vi "RestartIfDisconnected.vi"(8 "error in (no error)":errorcluster, 9 "connection timeout":i32=-1, 11 "NetworkStreamReader in":refnum<class "NetworkStreamReader.lvclass">) -> (0 "error out":errorcluster, 3 "NetworkStreamReader out":refnum<class "NetworkStreamReader.lvclass">)   [LabVIEW 2011, in "NetworkStreamReader.lvclass"]
uses:
  NetworkStreamReader.lvclass
  NetworkStreamReader.lvclass/NetworkStreamReader.ctl
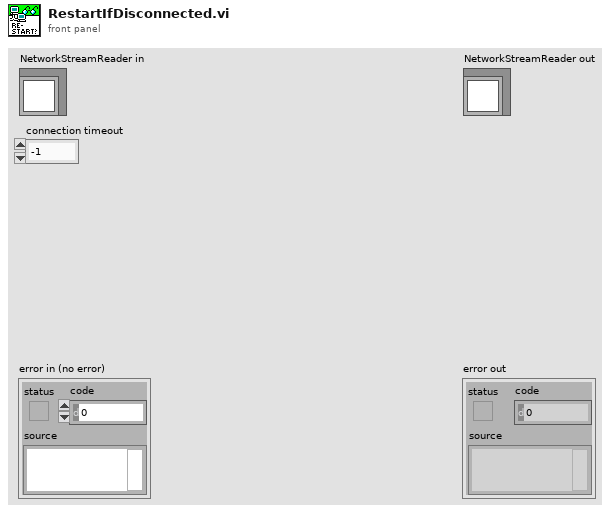
[diagram p1: front panel]
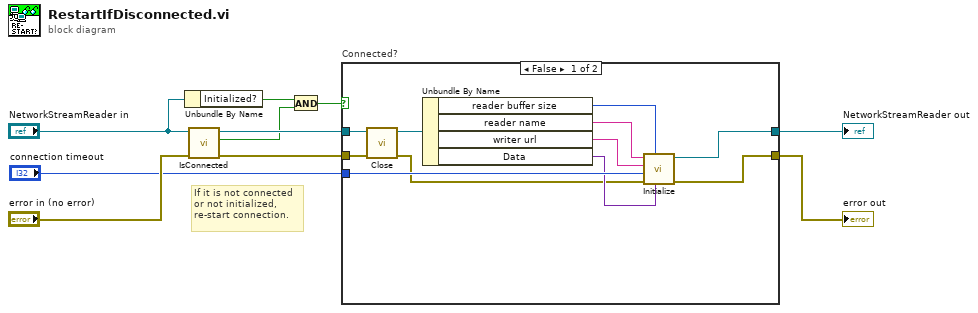
[diagram p0: block diagram]
diagram:
  # "If it is not connected\nor not initialized,\nre-start connection."
  n1 = Unbundle By Name("NetworkStreamReader in") -> ("Initialized?"=w2:bool)
  n2 = call "IsConnected.vi"("error in (no error)"="error in (no error)", "NetworkStreamReader in"="NetworkStreamReader in") -> ("error out"=w4:errorcluster, "Connected?"=w1:bool, "NetworkStreamReader out"=w5:refnum<class "NetworkStreamReader.lvclass">)  [unwired: 7 in]
  n3 = And(x=w2, y=w1) -> (x .and. y?=w3:bool)
  n4 = case "Connected?" shown="False" w3 {
    tunnel: w5 -> [w19 w23]
    tunnel: w4 -> [w18 w22]
    tunnel: [w12 w23] -> w7
    tunnel: [w11 w22] -> w9
    tunnel: "connection timeout" -> [w21 _]
    frame False {
      n5 = call "Close.vi"("error in (no error)"=w18, "NetworkStreamReader in"=w19) -> ("error out"=w13:errorcluster, "NetworkStreamReader out"=w17:refnum<class "NetworkStreamReader.lvclass">)  [unwired: 8 in]
      n6 = Unbundle By Name(w17) -> ("reader buffer size"=w20:i32, "reader name"=w16:string, "writer url"=w15:string, "Data"=w14:variant)
      n7 = call "Initialize.vi"("Default return"=w14, "reader buffer size"=w20, "error in (no error)"=w13, "connection timeout"=w21, "writer url"=w15, "reader name"=w16) -> ("error out"=w11:errorcluster, "NetworkStreamWriter out"=w12:refnum<class "NetworkStreamReader.lvclass">)  [unwired: 3 in, 1 out]
    }
    frame True {
    }
  }
  "error out" <- w9
  "NetworkStreamReader out" <- w7
